vi "n control command.vi"(7 "data":u16, 8 "error in (no error)":errorcluster, 9 "axis":u16, 10 "head":u16, 11 "n":u16) -> (0 "error out":errorcluster)   [LabVIEW 2015, in "SCANalone4x64.lvlib"]
doc: "__declspec(dllimport) void __stdcall n_control_command(unsigned short n, unsigned short head, unsigned short axis, unsigned short data);"
uses:
  <userlib>/SCANalone4x64/SCANalone4x64.lvlib
  <userlib>/SCANalone4x64/SCANalone4x64.dll
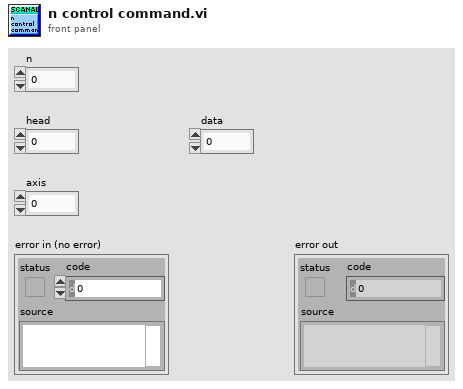
[diagram p1: front panel]
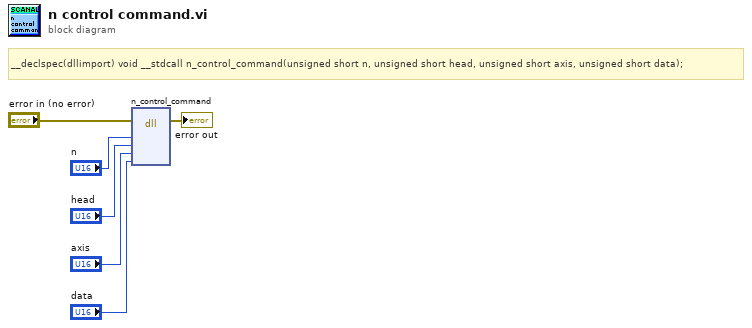
[diagram p0: block diagram]
diagram:
  # "__declspec(dllimport) void __stdcall n_control_command(unsigned short n, unsigned short head, unsigned short axis, unsigned short data);"
  n1 = dll-call lib="C:/Program Files/National Instruments/LabVIEW 2015/user.lib/SCANalone4x64/SCANalone4x64.*" fn="n_control_command"(error in="error in (no error)", "n"="n", "head"="head", "axis"="axis", "data"="data") -> (error out=→"error out":errorcluster)  [unwired: 7 in, 1 out]
